vi "HandleCollector.vi"(9 "Lower Collector?":bool, 10 "Raise Collector?":bool) -> (1 "CollectorEnum Input":T1)   [LabVIEW 2013]
doc: "Takes in two booleans of whether to raise or lower the collector, and the outpus the enum \"Raise\", \"Lower\", or \"Stop\""
uses:
  Autonomous/CollectorEnum.ctl
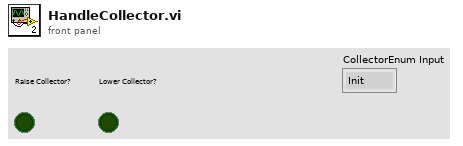
[diagram p1: front panel]
types:
  T1 = typedef "CollectorEnum.ctl" = enum16{"Init", "Raise", "Lower", "Stop", "GetStatus"}
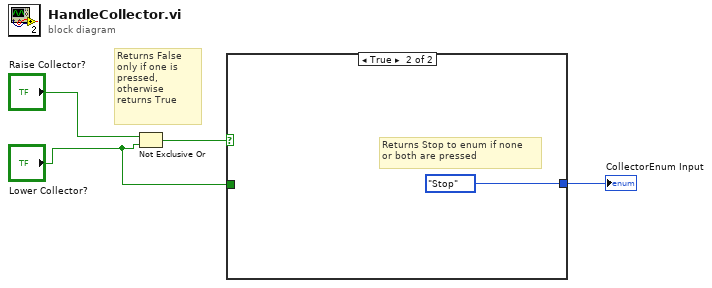
[diagram p0: block diagram]
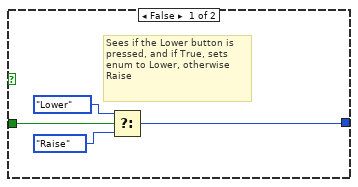
[diagram p2: hidden frame]
diagram:
  # "Returns False only if one is pressed, otherwise returns True"
  n1 = Not Exclusive Or(1:"Lower Collector?", 2:"Raise Collector?") -> (0:w3:bool)
  n2 = case shown="True" w3 {
    tunnel: [w5 CollectorEnum."Stop" ("Enum")] -> w4
    tunnel: "Lower Collector?" -> [w8 _]
    frame False {
      # "Sees if the Lower button is pressed, and if True, sets enum to Lower, otherwise Raise"
      n3 = Select(t=CollectorEnum."Lower" ("Enum"), s=w8, f=CollectorEnum."Raise" ("Enum")) -> (s? t:f=w5:T1)
    }
    frame True {
      # "Returns Stop to enum if none \nor both are pressed"
    }
  }
  "CollectorEnum Input" <- w4
